vi "关键参数交互.vi"(9 "量程下拉列表":refnum<vi>, 10 "测量模式下拉列表":refnum<vi>, 11 "参数下拉列表":refnum<vi>) -> ()   [LabVIEW 2016, in "斯坦道总磷.lvlib"]
panel:
  out "x != y?":T1
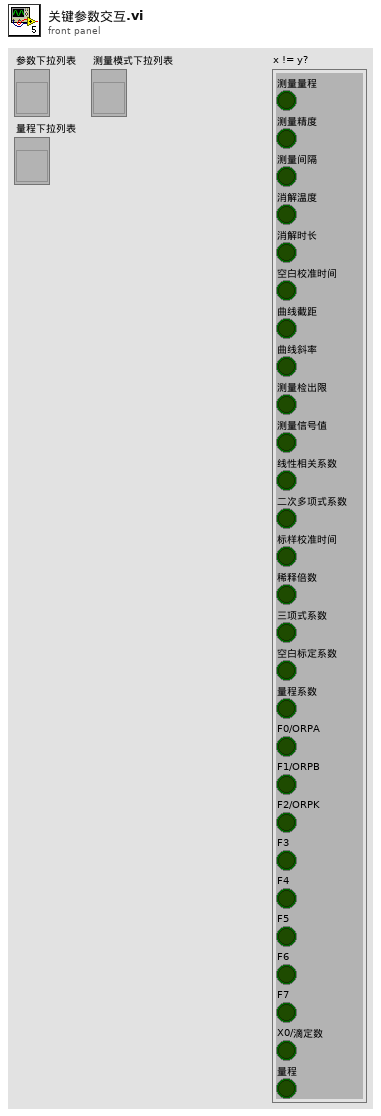
[diagram p1: front panel]
types:
  T1 = cluster{"测量量程":bool, "测量精度":bool, "测量间隔":bool, "消解温度":bool, "消解时长":bool, "空白校准时间":bool, "曲线截距":bool, "曲线斜率":bool, "测量检出限":bool, "测量信号值":bool, "线性相关系数":bool, "二次多项式系数":bool, "标样校准时间":bool, "稀释倍数":bool, "三项式系数":bool, "空白标定系数":bool, "量程系数":bool, "F0/ORPA":bool, "F1/ORPB":bool, "F2/ORPK":bool, "F3":bool, "F4":bool, "F5":bool, "F6":bool, "F7":bool, "X0/滴定数":bool, "量程":bool}
  T2 = cluster{"chose":string, "公式":cluster{"X^2":dbl, "X":dbl, "b":dbl}}
  T3 = cluster{"测量量程":dbl, "测量精度":dbl, "测量间隔":dbl, "消解温度":dbl, "消解时长":dbl, "空白校准时间":timestamp, "曲线截距":dbl, "曲线斜率":dbl, "测量检出限":dbl, "测量信号值":dbl, "线性相关系数":dbl, "二次多项式系数":dbl, "标样校准时间":timestamp, "稀释倍数":dbl, "三项式系数":dbl, "空白标定系数":dbl, "量程系数":dbl, "F0/ORPA":dbl, "F1/ORPB":dbl, "F2/ORPK":dbl, "F3":dbl, "F4":dbl, "F5":dbl, "F6":dbl, "F7":dbl, "X0/滴定数":dbl, "量程":dbl}
  T4 = cluster{"时间标识":timestamp, "设备":string, "日志信息":string, "流程参数":string}
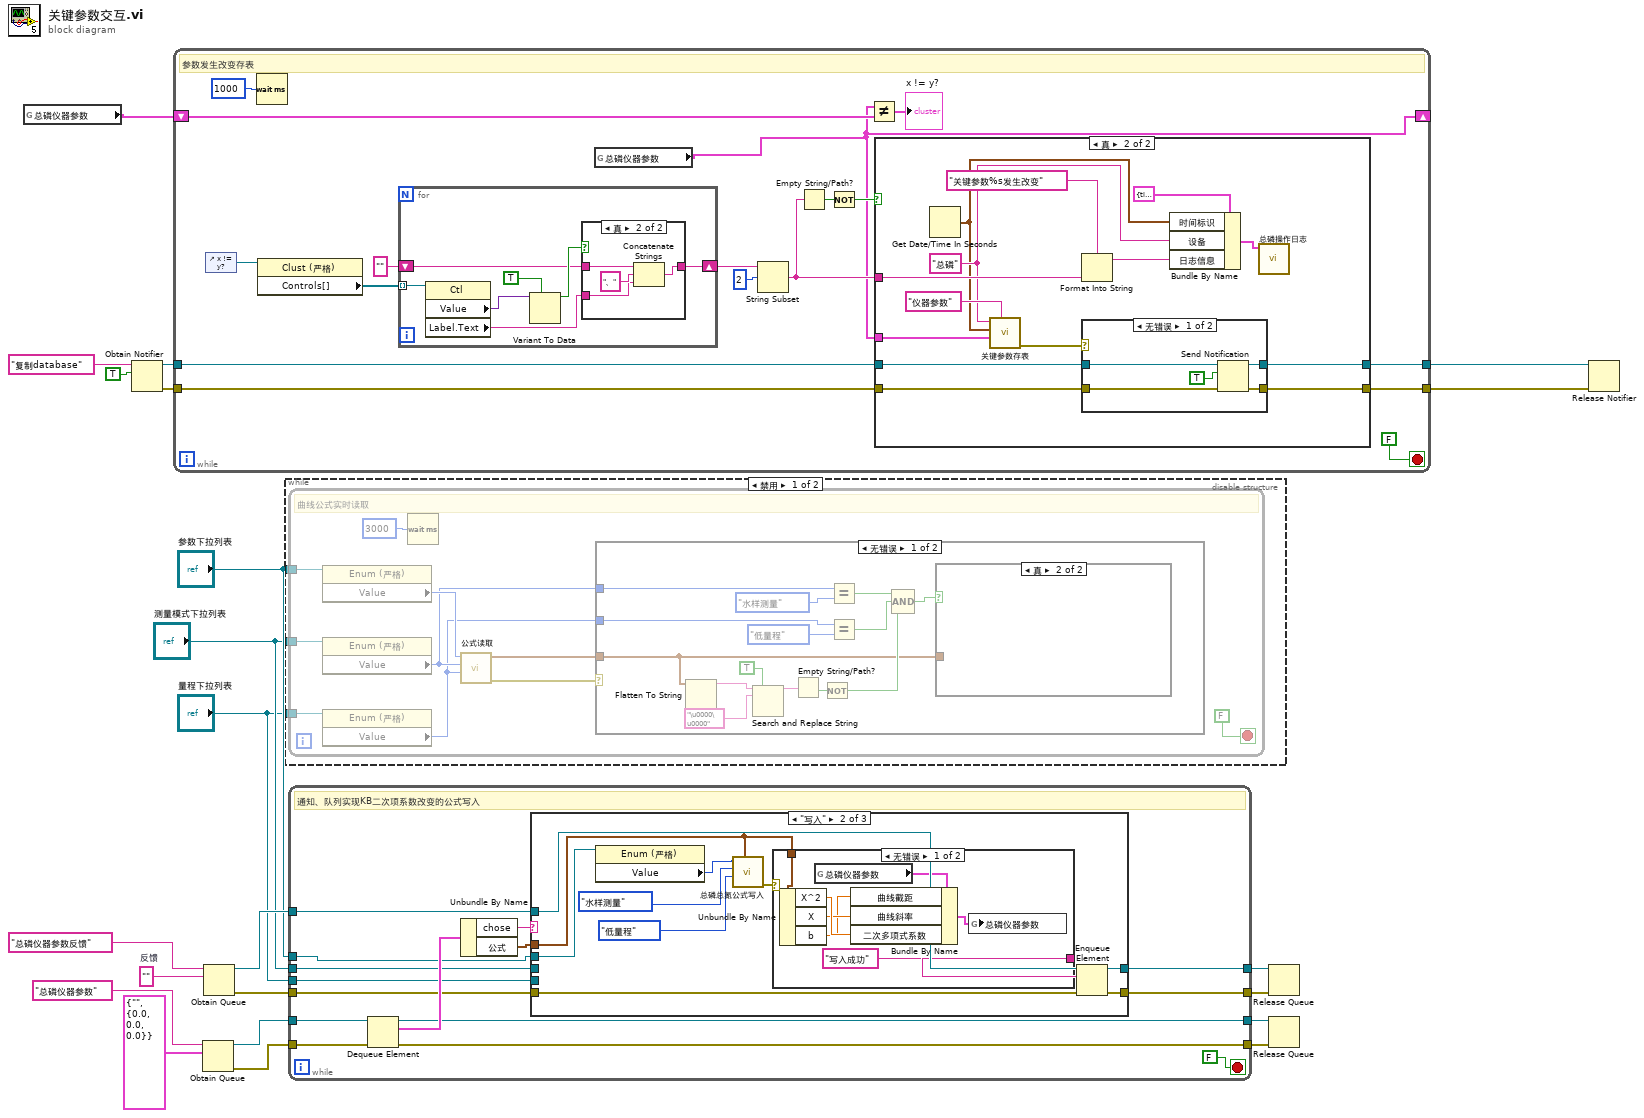
[diagram p0: block diagram]
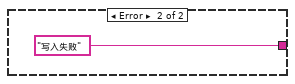
[diagram p6: hidden frame]
diagram:
  w16 = ""  # 反馈
  n1 = global read "总磷断电保存全局变量.vi" "总磷仪器参数"() -> (w1:T3)
  n2 = Obtain Notifier(name (unnamed)="复制database" ("名称（未命名）"), notification data type=TRUE) -> (notifier out=w5:refnum<notifier>, error out=w4:errorcluster)  [unwired: 2 in, 1 out]
  n3 = while {
    shift-right: [w23] -> _
    shift-left: w1 -> [w37]
    tunnel: w5 -> [w34]
    tunnel: w4 -> [w33]
    tunnel: [w32] -> w3
    tunnel: [w31] -> w2
    stop <- FALSE stop-if-true
    # "参数发生改变存表"
    n4 = control-ref of="x != y?"() -> (w35:refnum<vi>)
    n5 = Wait (ms)(milliseconds to wait=u32 1000 ("等待时间（毫秒）")) -> ()  [unwired: 1 out]
    n6 = property class="Clust (严格)"(reference=w35) -> ("Controls[]"=w27:refnum<vi>[])  [unwired: 1 in, 2 out]
    n7 = for {
      tunnel: w27 -> [w46] mode=indexing
      shift-right: [w40] -> w29
      shift-left: "" -> [w42]
      n8 = property class="Ctl"(reference=w46) -> ("Value"=w44:variant, "Label.Text"=w41:string)  [unwired: 1 in, 2 out]
      n9 = Variant To Data(type=TRUE, Variant=w44) -> (data=w43:bool)  [unwired: 1 in, 1 out]
      n10 = case shown="真" w43 {
        tunnel: w42 -> [w47 w51]
        tunnel: w41 -> [_ w48]
        tunnel: [w47 w50] -> w40
        frame False {
        }
        frame True {
          n11 = Concatenate Strings(w51, "、", w48) -> (w50:string)
        }
      }
    }
    n12 = global read "总磷断电保存全局变量.vi" "总磷仪器参数"() -> (w23:T3)
    n13 = String Subset(string=w29, offset (0)=2 ("偏移量(0)")) -> (substring=w24:string)  [unwired: 1 in]
    n14 = Empty String/Path?(string/path=w24) -> (empty?=w26:bool)
    n15 = Not(x=w26) -> (.not. x?=w25:bool)
    n16 = Not Equal?(x=w23, y=w37) -> (x != y?=→"x != y?":T1)
    n17 = case shown="真" w25 {
      tunnel: w23 -> [_ w55]
      tunnel: w24 -> [_ w65]
      tunnel: w34 -> [w53 w63]
      tunnel: w33 -> [w52 w62]
      tunnel: [w53 w61] -> w32
      tunnel: [w52 w60] -> w31
      frame False {
      }
      frame True {
        w57 = "总磷" ("仪器名称")
        n18 = Get Date/Time In Seconds() -> (seconds since 1Jan1904=w56:timestamp)
        n19 = call "关键参数存表.vi"("table"="仪器参数", "仪器参数"=w55, "datatime"=w56, "仪器名称"=w57) -> ("error out"=w54:errorcluster)  [unwired: 7 in]
        n20 = Format Into String(format string="关键参数%s发生改变" ("格式字符串"), w65) -> (resulting string=w64:string)  [unwired: 2 in, 1 out]
        n21 = case shown="无错误" w54 {
          tunnel: w63 -> [w72 w74]
          tunnel: w62 -> [w71 w73]
          tunnel: [w69 w74] -> w61
          tunnel: [w68 w73] -> w60
          frame No Error {
            n22 = Send Notification(notification=TRUE ("通知"), notifier=w72, error in (no error)=w71) -> (notifier out=w69:refnum<notifier>, error out=w68:errorcluster)
          }
          frame Error {
          }
        }
        n23 = Bundle By Name(cluster=T4 {"时间标识"=timestamp(0 s since 1904-01-01), "设备"="", "日志信息"="", "流程参数"=""} ("data in"), "时间标识"=w56, "设备"=w57, "日志信息"=w64) -> (w59:T4)
        n24 = call "总磷操作日志.vi"("data in"=w59) -> ()  [unwired: 11 in]
      }
    }
  }
  n25 = Obtain Queue(name (unnamed)="总磷仪器参数" ("名称（未命名）"), element data type=T2 {"chose"="", "公式"={"X^2"=0.0, "X"=0.0, "b"=0.0}}) -> (queue out=w12:refnum<queue>, error out=w11:errorcluster)  [unwired: 3 in, 1 out]
  n26 = Obtain Queue(name (unnamed)="总磷仪器参数反馈" ("名称（未命名）"), element data type=w16) -> (queue out=w17:refnum<queue>, error out=w15:errorcluster)  [unwired: 3 in, 1 out]
  n27 = disable-structure shown="禁用" {
    disable-tunnel: "参数下拉列表" -> [w77 _]
    disable-tunnel: "测量模式下拉列表" -> [w76 _]
    disable-tunnel: "量程下拉列表" -> [w75 _]
    frame Disabled {
      n28 = while {
        tunnel: w77 -> [w80]
        tunnel: w76 -> [w79]
        tunnel: w75 -> [w78]
        stop <- FALSE stop-if-true
        # "曲线公式实时读取"
        n29 = property class="Enum (严格)"(reference=w80) -> ("Value"=w85:enum16{"总磷", "总氮", "氨氮"})  [unwired: 1 in, 2 out]
        n30 = property class="Enum (严格)"(reference=w79) -> ("Value"=w83:enum16{"水样测量", "零点核查", "跨度核查", "标样核查", "加标回收"})  [unwired: 1 in, 2 out]
        n31 = property class="Enum (严格)"(reference=w78) -> ("Value"=w82:enum16{"低量程", "高量程"})  [unwired: 1 in, 2 out]
        n32 = Wait (ms)(milliseconds to wait=u32 3000 ("等待时间（毫秒）")) -> ()  [unwired: 1 out]
        n33 = call "公式读取.vi"("量程"=w82, "测量模式"=w83, "测量参数"=w85) -> ("error out"=w81:errorcluster, "公式"=w84:cluster{"X^2":dbl, "X":dbl, "b":dbl})  [unwired: 7 in]
        n34 = case shown="无错误" w81 {
          tunnel: w83 -> [w101 _]
          tunnel: w84 -> [w88 _]
          tunnel: w82 -> [w95 _]
          frame No Error {
            n35 = Flatten To String(anything=w88) -> (data string=w94:string)  [unwired: 3 in, 2 out]
            n36 = Search and Replace String(replace all?=TRUE ("替换全部？(F)"), input string=w94, search string="\u0000\u0000" ("数据字符串")) -> (result string=w93:string)  [unwired: 5 in, 3 out]
            n37 = Empty String/Path?(string/path=w93) -> (empty?=w92:bool)
            n38 = Not(x=w92) -> (.not. x?=w89:bool)
            n39 = Equal?(x=w101, y=enum16{"水样测量", "零点核查", "跨度核查", "标样核查", "加标回收"}."水样测量") -> (x = y?=w98:bool)
            n40 = Equal?(x=w95, y=enum16{"低量程", "高量程"}."低量程") -> (x = y?=w97:bool)
            n41 = Compound Arithmetic op=AND ("复合运算")(w98, w97, w89) -> (w96:bool)
            n42 = case shown="真" w96 {
              tunnel: w88 -> [_ _]
              frame False {
              }
              frame True {
              }
            }
          }
          frame Error {
          }
        }
      }
    }
    frame Enabled {
    }
  }
  n43 = while {
    tunnel: w12 -> [w115]
    tunnel: w11 -> [w114]
    tunnel: [w106] -> w20
    tunnel: [w105] -> w19
    tunnel: w17 -> [w110]
    tunnel: w15 -> [w109]
    tunnel: [w108] -> w14
    tunnel: [w107] -> w13
    tunnel: "参数下拉列表" -> [w104]
    tunnel: "测量模式下拉列表" -> [w103]
    tunnel: "量程下拉列表" -> [w102]
    stop <- FALSE stop-if-true
    # "通知、队列实现KB二次项系数改变的公式写入"
    n44 = Dequeue Element(queue=w115, error in (no error)=w114) -> (queue out=w106:refnum<queue>, element=w113:T2, error out=w105:errorcluster)  [unwired: 1 in, 1 out]
    n45 = Unbundle By Name(w113) -> ("chose"=w112:string, "公式"=w111:cluster{"X^2":dbl, "X":dbl, "b":dbl})
    n46 = case shown="\"写入\"" w112 {
      tunnel: w111 -> [_ w123 _]
      tunnel: w110 -> [w118 w129 w139]
      tunnel: w109 -> [w117 w127 w138]
      tunnel: [w118 w126 w139] -> w108
      tunnel: [w117 w125 w138] -> w107
      tunnel: w104 -> [_ w124 _]
      tunnel: w103 -> [_ _ _]
      tunnel: w102 -> [_ _ _]
      frame "假", Default {
      }
      frame "写入" {
        n47 = property class="Enum (严格)"(reference=w124) -> ("Value"=w122:enum16{"总磷", "总氮", "氨氮"})  [unwired: 1 in, 2 out]
        n48 = call "总磷总氮公式写入.vi"("公式"=w123, "量程"=enum16{"低量程", "高量程"}."低量程", "测量模式"=enum16{"水样测量", "零点核查", "跨度核查", "标样核查", "加标回收"}."水样测量", "测量参数"=w122) -> ("error out"=w119:errorcluster)  [unwired: 7 in]
        n49 = case shown="无错误" w119 {
          tunnel: ["写入成功" ("消息") "写入失败" ("消息")] -> w128
          tunnel: w123 -> [w135 _]
          frame No Error {
            n50 = Unbundle By Name(w135) -> ("X^2"=w134:dbl, "X"=w133:dbl, "b"=w132:dbl)
            n51 = global read "总磷断电保存全局变量.vi" "总磷仪器参数"() -> (w130:T3)
            n52 = Bundle By Name(cluster=w130, "曲线截距"=w132, "曲线斜率"=w133, "二次多项式系数"=w134) -> (w131:T3)
            n53 = global write "总磷断电保存全局变量.vi" "总磷仪器参数"(w131) -> ()
          }
          frame Error {
          }
        }
        n54 = Enqueue Element(queue=w129, element=w128, error in (no error)=w127) -> (queue out=w126:refnum<queue>, error out=w125:errorcluster)  [unwired: 1 in, 1 out]
      }
      frame "读取" {
      }
    }
  }
  n55 = Release Queue(queue=w14, error in (no error)=w13) -> ()  [unwired: 1 in, 3 out]
  n56 = Release Queue(queue=w20, error in (no error)=w19) -> ()  [unwired: 1 in, 3 out]
  n57 = Release Notifier(notifier=w3, error in (no error)=w2) -> ()  [unwired: 1 in, 3 out]
